vi "get_build_specs.vi"(8 "error in (no error)":errorcluster, 11 "project path":path) -> (0 "error out":errorcluster, 3 "build_spec_info []":T1[](array[typedef]))   [LabVIEW 2015, in "lv-build.lvlib"]
uses:
  lv-build.lvlib
  _controls/build_specification.ctl
  _controls/build_type.ctl
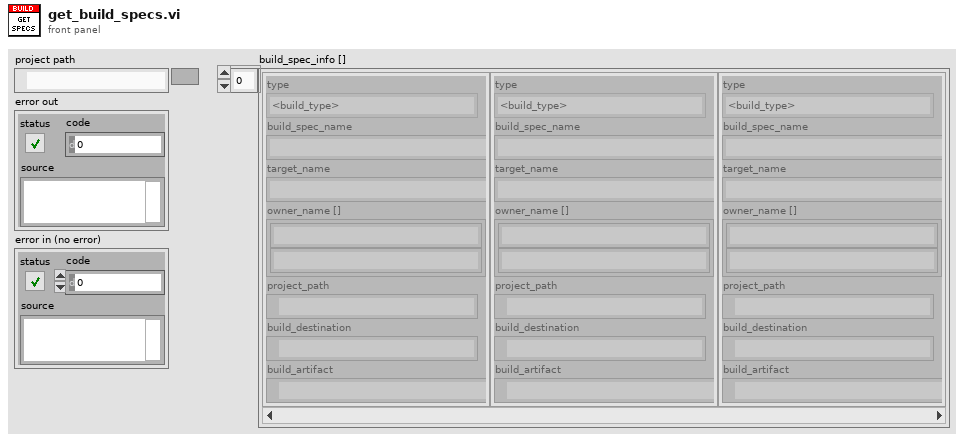
[diagram p1: front panel]
types:
  T1 = typedef "lv-build.lvlib/build_specification.ctl" = cluster{"type":T2, "build_spec_name":string, "target_name":string, "owner_name []":string[], "project_path":path, "build_destination":path, "build_artifact":path}
  T2 = typedef "lv-build.lvlib/build_type.ctl" = enum16{"<build_type>", "application_pc", "application_rt", "installer", "llb", "lvlibp", "zip", "fpga", "<null>"}
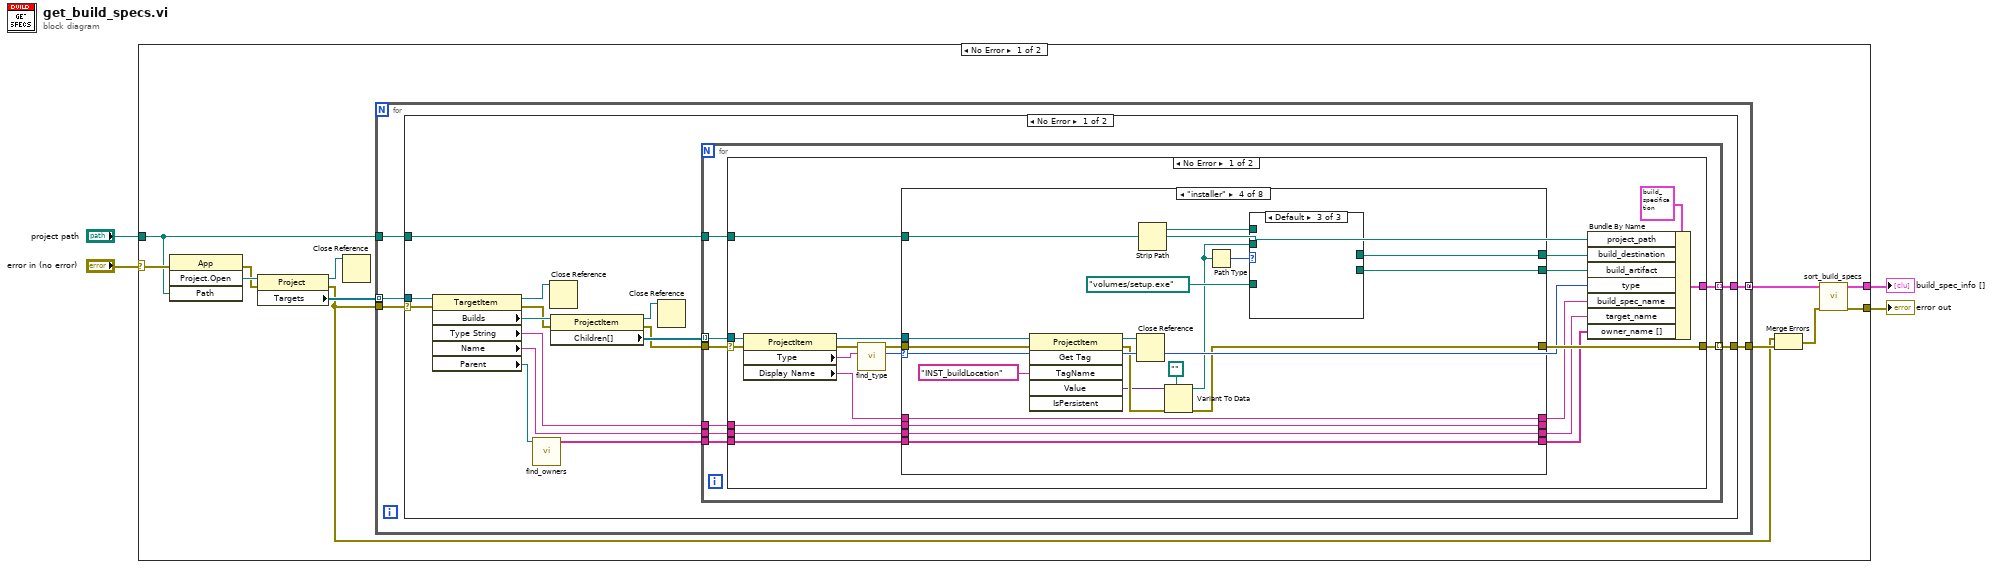
[diagram p0: block diagram]
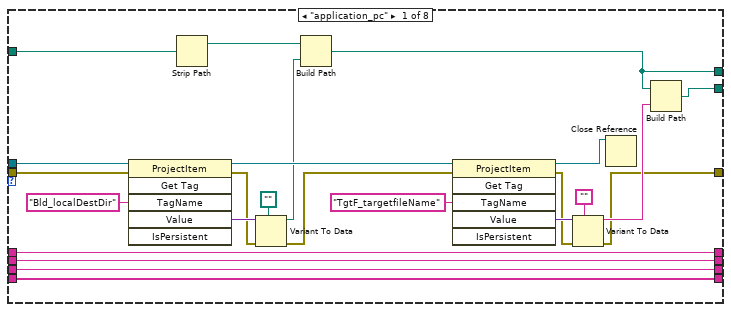
[diagram p2: hidden frame]
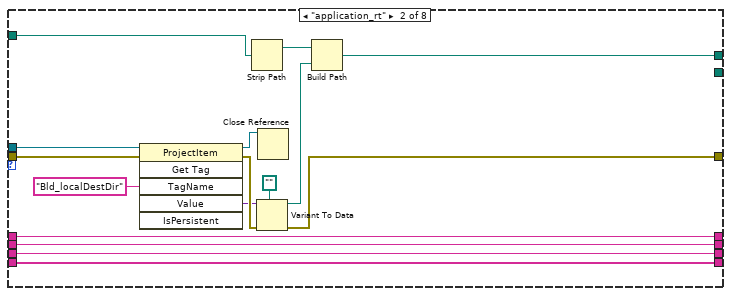
[diagram p3: hidden frame]
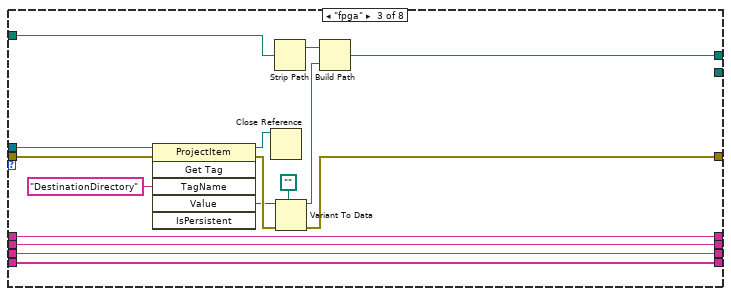
[diagram p4: hidden frame]
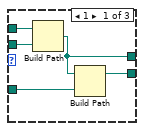
[diagram p5: hidden frame]
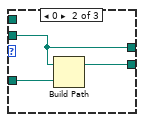
[diagram p6: hidden frame]
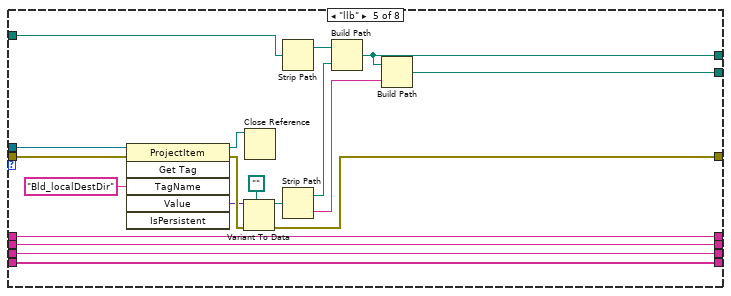
[diagram p7: hidden frame]
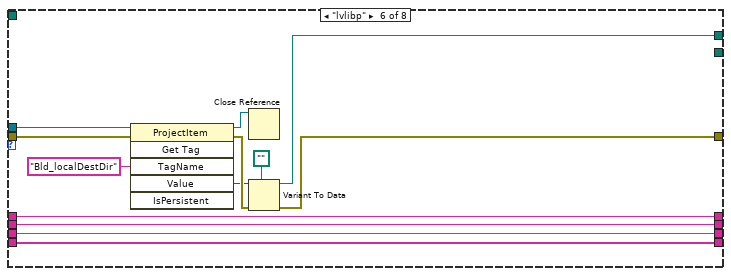
[diagram p8: hidden frame]
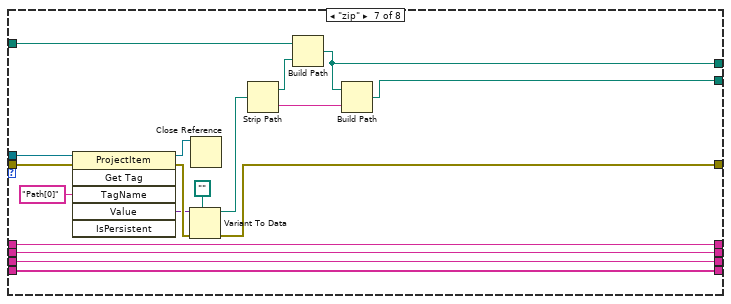
[diagram p9: hidden frame]
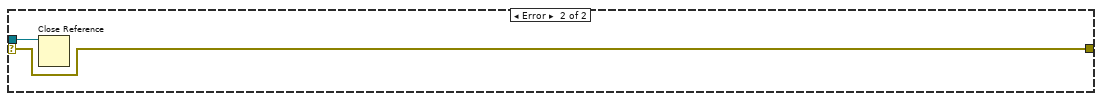
[diagram p11: hidden frame]
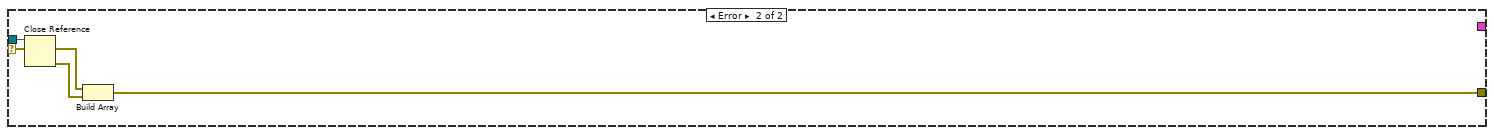
[diagram p12: hidden frame]
diagram:
  n1 = case shown="No Error" "error in (no error)" {
    selector: "error in (no error)" -> [w11 w205]
    tunnel: [w12 w205] -> w3
    tunnel: [w14 _] -> w2
    tunnel: "project path" -> [w7 _]
    frame No Error {
      n2 = invoke class="App" method="Project.Open"(error in=w11, "Path"=w7) -> (error out=w8:errorcluster, "Project:Open"=w10:refnum<vi>)  [unwired: 2 in, 2 out]
      n3 = property class="Project"(reference=w10, error in=w8) -> (reference out=w5:refnum<vi>, error out=w6:errorcluster, "Targets"=w9:refnum<vi>[])
      n4 = Close Reference(reference=w5) -> ()  [unwired: 1 in, 1 out]
      n5 = for {
        tunnel: w9 -> [w21] mode=indexing
        tunnel: w7 -> [w18]
        tunnel: w6 -> [w20]
        tunnel: [w19] -> w16
        tunnel: [w17] -> w15 mode=concatenating
        n6 = case shown="No Error" w20 {
          selector: w20 -> [w36 w203]
          tunnel: w21 -> [w34 w204]
          tunnel: [w33 w202] -> w19
          tunnel: w18 -> [w28 _]
          tunnel: [w26 _] -> w17
          frame No Error {
            n7 = property class="TargetItem"(reference=w34, error in=w36) -> (reference out=w32:refnum<vi>, error out=w23:errorcluster, "Builds"=w35:refnum<vi>, "Type String"=w27:string, "Name"=w29:string, "Parent"=w25:refnum<vi>)
            n8 = call "find_owners.vi"("owner"=w25) -> ("owner_name []"=w24:string[])  [unwired: 9 in, 1 out]
            n9 = Close Reference(reference=w32) -> ()  [unwired: 1 in, 1 out]
            n10 = property class="ProjectItem"(reference=w35, error in=w23) -> (reference out=w31:refnum<vi>, error out=w22:errorcluster, "Children[]"=w30:refnum<vi>[])
            n11 = Close Reference(reference=w31) -> ()  [unwired: 1 in, 1 out]
            n12 = for {
              tunnel: w30 -> [w42] mode=indexing
              tunnel: w29 -> [w41]
              tunnel: w28 -> [w40]
              tunnel: w22 -> [w43]
              tunnel: [w44] -> w33 mode=indexing
              tunnel: w27 -> [w39]
              tunnel: [w38] -> w26 mode=indexing
              tunnel: w24 -> [w37]
              n13 = case shown="No Error" w43 {
                selector: w43 -> [w63 w199]
                tunnel: [w64 w199] -> w44
                tunnel: w42 -> [w61 w200]
                tunnel: w41 -> [w50 _]
                tunnel: w40 -> [w57 _]
                tunnel: w39 -> [w51 _]
                tunnel: [w54 _] -> w38
                tunnel: w37 -> [w47 _]
                frame No Error {
                  n14 = property class="ProjectItem"(reference=w61, error in=w63) -> (reference out=w62:refnum<vi>, error out=w60:errorcluster, "Type"=w58:string, "Display Name"=w52:string)
                  n15 = call "find_type.vi"("type_string"=w58, "error in (no error)"=w60) -> ("type_enum"=w53:T2, "error out"=w59:errorcluster)  [unwired: 8 in]
                  n16 = case shown="\"installer\"" w53 {
                    tunnel: [w66 w100 w117 w133 w161 w172 w192 w198] -> w64
                    tunnel: [w70 w95 w109 w123 w150 w173 w182 _] -> w55
                    tunnel: w59 -> [w88 w104 w120 w138 w166 w178 w197 w198]
                    tunnel: w62 -> [w79 w98 w116 w139 w160 w179 w190 _]
                    tunnel: w57 -> [w74 w97 w112 w131 w158 _ w189 _]
                    tunnel: w52 -> [w82 w91 w108 w128 w152 w168 w184 _]
                    tunnel: w51 -> [w83 w92 w107 w129 w153 w169 w185 _]
                    tunnel: w50 -> [w84 w93 w106 w130 w154 w170 w186 _]
                    tunnel: [w82 w91 w108 w128 w152 w168 w184 _] -> w49
                    tunnel: [w83 w92 w107 w129 w153 w169 w185 _] -> _
                    tunnel: [w84 w93 w106 w130 w154 w170 w186 _] -> w48
                    tunnel: w47 -> [w81 w90 w105 w127 w151 w167 w183 _]
                    tunnel: [w81 w90 w105 w127 w151 w167 w183 _] -> w46
                    tunnel: [w72 _ _ w125 w148 _ w180 _] -> w45
                    frame "application_pc" {
                      n17 = invoke class="ProjectItem" method="Get Tag"(reference=w79, error in=w88, "TagName"="Bld_localDestDir" ("Tag Name")) -> (reference out=w78:refnum<vi>, error out=w69:errorcluster, "Value"=w86:variant)  [unwired: 3 in, 3 out]
                      n18 = Strip Path(path=w74) -> (stripped path=w65:path)  [unwired: 1 out]
                      n19 = Variant To Data(error in=w69, type=path "", Variant=w86) -> (data=w71:path, error out=w68:errorcluster)
                      n20 = Build Path(base path=w65, name or relative path=w71) -> (appended path=w70:path)
                      n21 = invoke class="ProjectItem" method="Get Tag"(reference=w78, error in=w68, "TagName"="TgtF_targetfileName" ("Tag Name")) -> (reference out=w75:refnum<vi>, error out=w67:errorcluster, "Value"=w77:variant)  [unwired: 3 in, 3 out]
                      n22 = Variant To Data(error in=w67, type="", Variant=w77) -> (data=w73:string, error out=w66:errorcluster)
                      n23 = Close Reference(reference=w75) -> ()  [unwired: 1 in, 1 out]
                      n24 = Build Path(base path=w70, name or relative path=w73) -> (appended path=w72:path)
                    }
                    frame "application_rt" {
                      n25 = invoke class="ProjectItem" method="Get Tag"(reference=w98, error in=w104, "TagName"="Bld_localDestDir" ("Tag Name")) -> (reference out=w103:refnum<vi>, error out=w102:errorcluster, "Value"=w101:variant)  [unwired: 3 in, 3 out]
                      n26 = Strip Path(path=w97) -> (stripped path=w94:path)  [unwired: 1 out]
                      n27 = Variant To Data(error in=w102, type=path "", Variant=w101) -> (data=w96:path, error out=w100:errorcluster)
                      n28 = Close Reference(reference=w103) -> ()  [unwired: 1 in, 1 out]
                      n29 = Build Path(base path=w94, name or relative path=w96) -> (appended path=w95:path)
                    }
                    frame "fpga" {
                      n30 = invoke class="ProjectItem" method="Get Tag"(reference=w116, error in=w120, "TagName"="DestinationDirectory" ("Tag Name")) -> (reference out=w119:refnum<vi>, error out=w118:errorcluster, "Value"=w113:variant)  [unwired: 3 in, 3 out]
                      n31 = Close Reference(reference=w119) -> ()  [unwired: 1 in, 1 out]
                      n32 = Strip Path(path=w112) -> (stripped path=w111:path)  [unwired: 1 out]
                      n33 = Variant To Data(error in=w118, type=path "", Variant=w113) -> (data=w110:path, error out=w117:errorcluster)
                      n34 = Build Path(base path=w111, name or relative path=w110) -> (appended path=w109:path)
                    }
                    frame "installer" {
                      n35 = invoke class="ProjectItem" method="Get Tag"(reference=w139, error in=w138, "TagName"="INST_buildLocation" ("Tag Name")) -> (reference out=w137:refnum<vi>, error out=w135:errorcluster, "Value"=w134:variant)  [unwired: 3 in, 3 out]
                      n36 = Close Reference(reference=w137) -> ()  [unwired: 1 in, 1 out]
                      n37 = Strip Path(path=w131) -> (stripped path=w124:path)  [unwired: 1 out]
                      n38 = Variant To Data(error in=w135, type=path "", Variant=w134) -> (data=w122:path, error out=w133:errorcluster)
                      n39 = Path Type(1:w122) -> (0:w121:i16)
                      n40 = case shown="Default" w121 {
                        tunnel: path "volumes/setup.exe" ("appended path") -> [w144 w147 _]
                        tunnel: [w143 w146 _] -> w125
                        tunnel: w124 -> [w142 _ _]
                        tunnel: [w141 w145 _] -> w123
                        tunnel: w122 -> [w140 w145 _]
                        frame 1 {
                          n41 = Build Path(base path=w142, name or relative path=w140) -> (appended path=w141:path)
                          n42 = Build Path(base path=w141, name or relative path=w144) -> (appended path=w143:path)
                        }
                        frame 0 {
                          n43 = Build Path(base path=w145, name or relative path=w147) -> (appended path=w146:path)
                        }
                        frame Default {
                        }
                      }
                    }
                    frame "llb" {
                      n44 = invoke class="ProjectItem" method="Get Tag"(reference=w160, error in=w166, "TagName"="Bld_localDestDir" ("Tag Name")) -> (reference out=w165:refnum<vi>, error out=w163:errorcluster, "Value"=w162:variant)  [unwired: 3 in, 3 out]
                      n45 = Variant To Data(error in=w163, type=path "", Variant=w162) -> (data=w156:path, error out=w161:errorcluster)
                      n46 = Close Reference(reference=w165) -> ()  [unwired: 1 in, 1 out]
                      n47 = Strip Path(path=w158) -> (stripped path=w157:path)  [unwired: 1 out]
                      n48 = Strip Path(path=w156) -> (stripped path=w155:path, name=w149:string)
                      n49 = Build Path(base path=w157, name or relative path=w155) -> (appended path=w150:path)
                      n50 = Build Path(base path=w150, name or relative path=w149) -> (appended path=w148:path)
                    }
                    frame "lvlibp" {
                      n51 = invoke class="ProjectItem" method="Get Tag"(reference=w179, error in=w178, "TagName"="Bld_localDestDir" ("Tag Name")) -> (reference out=w177:refnum<vi>, error out=w175:errorcluster, "Value"=w174:variant)  [unwired: 3 in, 3 out]
                      n52 = Close Reference(reference=w177) -> ()  [unwired: 1 in, 1 out]
                      n53 = Variant To Data(error in=w175, type=path "", Variant=w174) -> (data=w173:path, error out=w172:errorcluster)
                    }
                    frame "zip" {
                      n54 = invoke class="ProjectItem" method="Get Tag"(reference=w190, error in=w197, "TagName"="Path[0]" ("Tag Name")) -> (reference out=w196:refnum<vi>, error out=w194:errorcluster, "Value"=w193:variant)  [unwired: 3 in, 3 out]
                      n55 = Variant To Data(error in=w194, type=path "", Variant=w193) -> (data=w188:path, error out=w192:errorcluster)
                      n56 = Close Reference(reference=w196) -> ()  [unwired: 1 in, 1 out]
                      n57 = Strip Path(path=w188) -> (stripped path=w187:path, name=w181:string)
                      n58 = Build Path(base path=w189, name or relative path=w187) -> (appended path=w182:path)
                      n59 = Build Path(base path=w182, name or relative path=w181) -> (appended path=w180:path)
                    }
                    frame Default {
                    }
                  }
                  n60 = Bundle By Name(cluster=T1 {"type"=enum."<build_type>", "build_spec_name"="", "target_name"="", "owner_name []"=[], "project_path"=path "", "build_destination"=path "", "build_artifact"=path ""} ("build spec path"), "project_path"=w57, "build_destination"=w55, "build_artifact"=w45, "type"=w53, "build_spec_name"=w49, "target_name"=w48, "owner_name []"=w46) -> (w54:T1)
                }
                frame Error {
                  n61 = Close Reference(reference=w200) -> ()  [unwired: 1 in, 1 out]
                }
              }
            }
          }
          frame Error {
            n62 = Close Reference(reference=w204) -> (error out=w201:errorcluster)  [unwired: 1 in]
            n63 = Build Array(w203, w201) -> (w202:errorcluster[])
          }
        }
      }
      n64 = Merge Errors(w6, w16) -> (w13:errorcluster)
      n65 = call "sort_build_specs.vi"("error in (no error)"=w13, "build_specifications in"=w15) -> ("error out"=w12:errorcluster, "build_specifications out"=w14:T1[])  [unwired: 8 in]
    }
    frame Error {
    }
  }
  "error out" <- w3
  "build_spec_info []" <- w2
